vi "Mod_OFDM_Get_Sub_Carrier_Selection.vi"(0 "Configure Variant":variant, 7 "Attribute Data Types":T2={"Pulse Shaping"={"System Filter"={"TX Filter"=enum."none", "Alpha"=0.0, "filter length"=0}, "Modulation system parameters"={"samples per symbol (16)"=0}, "symbol rate (Hz)"=0.0}, "FRAME Table"=[], "OFDM Frame"=[], "Sub Carrier Selection"={"Sub Carrier Selection"=[], "OFDM Parameters"={"# of Sub Carrier"=0, "Length Of Cylic Prefix"=0}}, "Symbol Table"=[], "Symbol Pool"=[], "Pool of Modulators"=[], "Pool of Data Sources"=[], "Atribute Names"={"Data Source Pool"="Data Source Pool ", "Modulator Source Pool"="Modulator Source Pool ", "OFDM SYMBOL POOL"="OFDM SYMBOL POOL", "Symbol Table"="Symbol Table", "Sub Carrier Selection"="Sub Carrier Selection", "OFDM Frame"="OFDM Frame", "FRAME Table"="FRAME Table", "Pulse Shaping"="Pulse Shaping"}} {"Pool of Data Sources"."Register Initial State" format="%08x"; "Pulse Shaping"."symbol rate (Hz)" min=1.0 step=1.0 format="%.2p"; "Pulse Shaping"."Modulation system parameters"."samples per symbol (16)" step=2; "Pulse Shaping"."System Filter"."Alpha" min=0.0 max=1.0 step=0.05 format="%.2f"}, 11 "error in":errorcluster) -> (4 "Configure Variant":variant, 6 "Sub Carrier Selection":string, 8 "Sub Carrier Selection":T1, 15 "error out":errorcluster)   [LabVIEW 2010]
uses:
  Controls(Type_DEf)/Attribute Data Types.ctl
  Controls(Type_DEf)/Configure Pulse Shaping.ctl
  Controls(Type_DEf)/Pool of Modulator Control.ctl
  Controls(Type_DEf)/Pool of Data Source Control.ctl
  Controls(Type_DEf)/Attribute Names.ctl
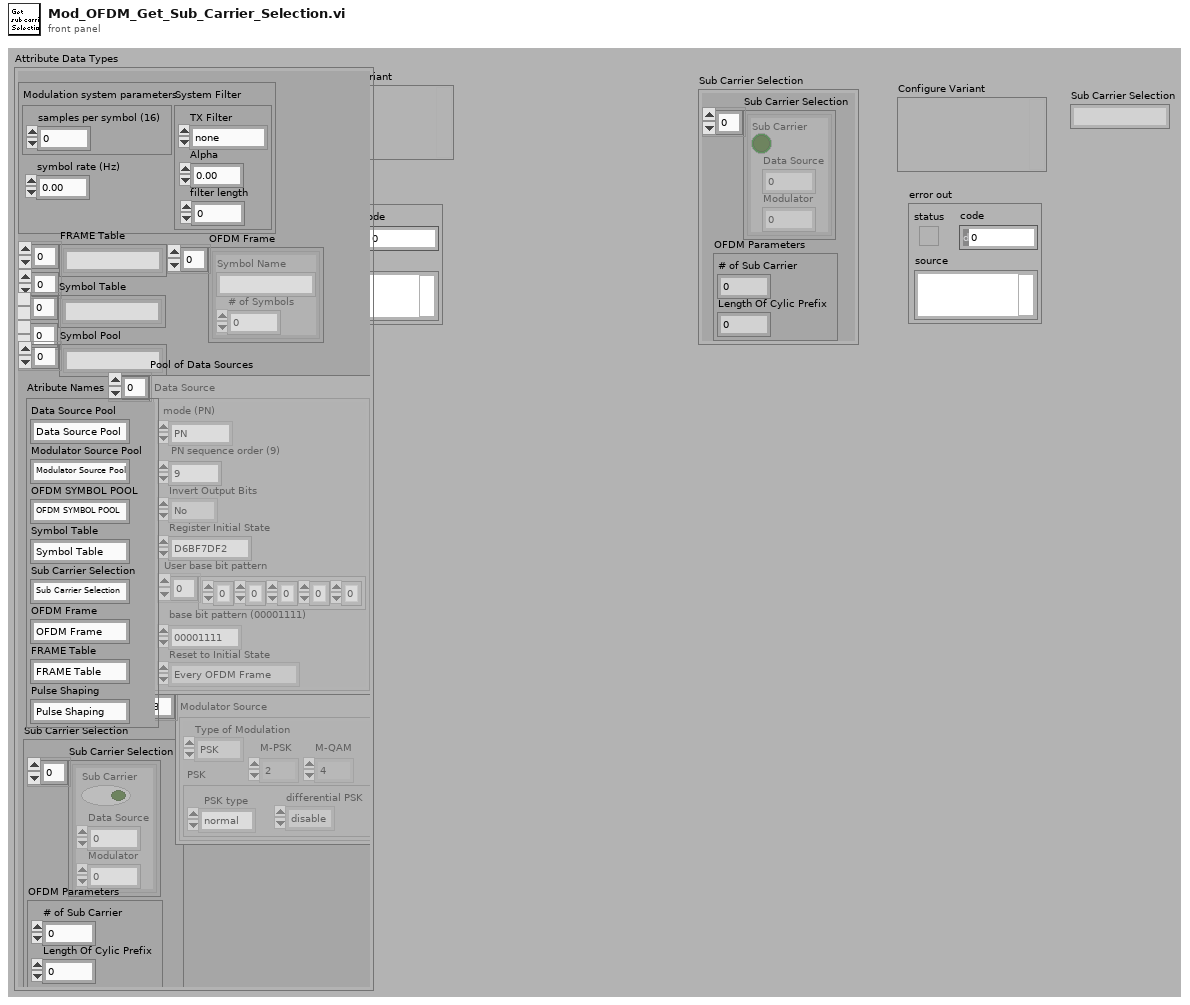
[diagram p1: front panel]
types:
  T1 = cluster{"Sub Carrier Selection":cluster{"Sub Carrier":bool, "Data Source":u16, "Modulator":u16}[], "OFDM Parameters":cluster{"# of Sub Carrier":i32, "Length Of Cylic Prefix":i32}}
  T2 = typedef "Attribute Data Types.ctl" = cluster{"Pulse Shaping":T3, "FRAME Table":string[][], "OFDM Frame":cluster{"Symbol Name":string, "# of Symbols":i32}[], "Sub Carrier Selection":cluster{"Sub Carrier Selection":cluster{"Sub Carrier":bool, "Data Source":u16, "Modulator":u16}[], "OFDM Parameters":cluster{"# of Sub Carrier":i32, "Length Of Cylic Prefix":i32}}, "Symbol Table":string[][], "Symbol Pool":string[], "Pool of Modulators":T4, "Pool of Data Sources":T5, "Atribute Names":T6}
  T3 = typedef "Configure Pulse Shaping.ctl" = cluster{"System Filter":cluster{"TX Filter":enum16{"none", "Raised Cosine", "Root Raised Cos"}, "Alpha":dbl, "filter length":i32}, "Modulation system parameters":cluster{"samples per symbol (16)":u32}, "symbol rate (Hz)":dbl}
  T4 = typedef "Pool of Modulator Control.ctl" = cluster{"M-QAM":enum16{"4", "16", "64", "256"}, "M-PSK":enum16{"2", "4", "8", "16", "32", "64", "128", "256"}, "Type of Modulation":enum16{"PSK", "QAM"}, " PSK":cluster{"differential PSK":enum16{"disable", "enable"}, "PSK type":enum16{"normal", "shifted", "offset"}}}[]
  T5 = typedef "Pool of Data Source Control.ctl" = cluster{"mode (PN)":enum16{"PN", "pattern", "user"}, "PN sequence order (9)":i32, "Invert Output Bits":enum16{"No", "Yes"}, "Register Initial State ":u32, "User base bit pattern":i8[], "base bit pattern (00001111)":enum16{"0", "1", "01", "0011", "00001111"}, "Reset to Initial State":enum16{"Every OFDM Frame", "Every OFDM Symbol", "Every Sub Carrier"}}[]
  T6 = typedef "Attribute Names.ctl" = cluster{"Data Source Pool":string, "Modulator Source Pool":string, "OFDM SYMBOL POOL":string, "Symbol Table":string, "Sub Carrier Selection":string, "OFDM Frame":string, "FRAME Table":string, "Pulse Shaping":string}
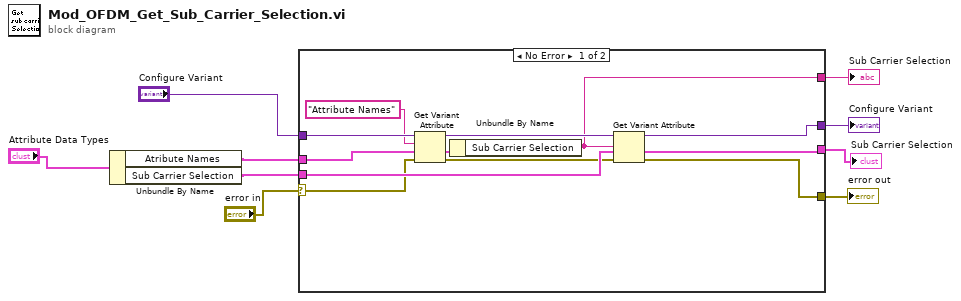
[diagram p0: block diagram]
diagram:
  n1 = Unbundle By Name("Attribute Data Types") -> ("Atribute Names"=w4:T6, "Sub Carrier Selection"=w3:T1)
  n2 = case shown="No Error" "error in" {
    selector: "error in" -> [w17 w22]
    tunnel: [w21 w22] -> w8
    tunnel: "Configure Variant" -> [w14 _]
    tunnel: [w20 _] -> w6
    tunnel: w4 -> [w13 _]
    tunnel: w3 -> [w19 _]
    tunnel: [w18 _] -> w2
    tunnel: [w10 _] -> w1
    frame No Error {
      n3 = Get Variant Attribute(Variant=w14, name="Attribute Names", default value (empty Variant)=w13, error in=w17) -> (duplicate Variant=w15:variant, value=w11:T6, error out=w16:errorcluster)  [unwired: 1 out]
      n4 = Unbundle By Name(w11) -> ("Sub Carrier Selection"=w10:string)
      n5 = Get Variant Attribute(Variant=w15, name=w10, default value (empty Variant)=w19, error in=w16) -> (duplicate Variant=w20:variant, value=w18:T1, error out=w21:errorcluster)  [unwired: 1 out]
    }
    frame Error {
    }
  }
  "error out" <- w8
  "Configure Variant" <- w6
  "Sub Carrier Selection" <- w2
  "Sub Carrier Selection" <- w1
